vi "Cut-Out File Manager.vi"(6 "Local Data in":T1, 7 ".ini Controller":enum16{"Read", "Write"}(ring), 8 "error in (no error)":errorcluster, 11 "Run Path":path) -> (0 "error out":errorcluster, 4 "Local Data out":T1)   [LabVIEW 2024]
uses:
  Controls/Local Data.ctl
  Controls/Test Cluster.ctl
  Controls/Excluded Information.ctl
  Controls/Language.ctl
  <vilib>/Utility/file.llb/Write Delimited Spreadsheet (string).vi
  <vilib>/Utility/file.llb/Read Delimited Spreadsheet (string).vi
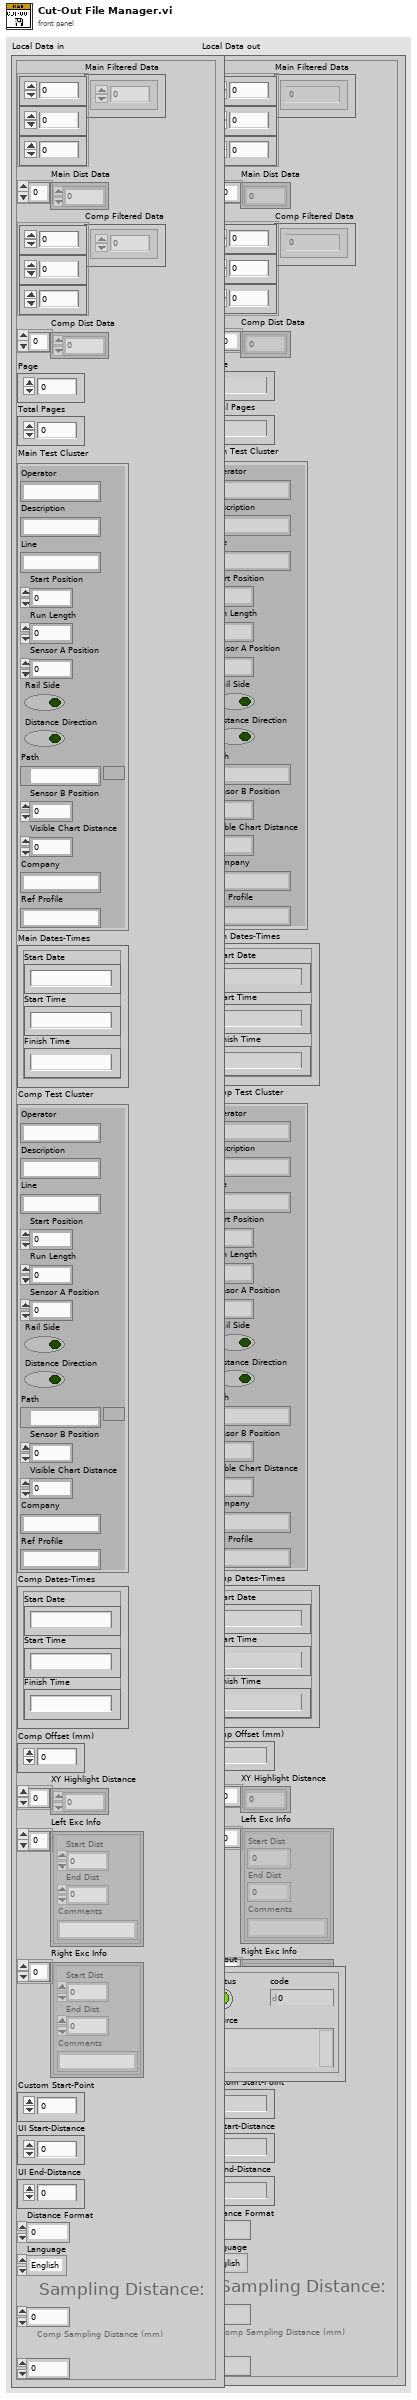
[diagram p1: front panel]
types:
  T1 = typedef "Local Data.ctl" = cluster{"Main Filtered Data":dbl[][][], "Main Dist Data":dbl[], "Comp Filtered Data":dbl[][][], "Comp Dist Data":dbl[], "Page":u8, "Total Pages":u8, "Main Test Cluster":T2, "Main Dates-Times":cluster{"Start Date":string, "Start Time":string, "Finish Time":string}, "Comp Test Cluster":T2, "Comp Dates-Times":cluster{"Start Date":string, "Start Time":string, "Finish Time":string}, "Comp Offset (mm)":i64, "XY Highlight Distance":dbl[], "Left Exc Info":T3[], "Right Exc Info":T3[], "Custom Start-Point":dbl, "UI Start-Distance":dbl, "UI End-Distance":dbl, "Distance Format":u8, "Language":T4, "Main Sampling Distance (mm)":dbl, "Comp Sampling Distance (mm)":dbl}
  T2 = typedef "Test Cluster.ctl" = cluster{"Operator":string, "Description":string, "Line":string, "Start Position":dbl, "Run Length":dbl, "Sensor A Position":dbl, "Rail Side":bool, "Distance Direction":bool, "Path":path, "Sensor B Position":dbl, "Visible Chart Distance":dbl, "Company":string, "Ref Profile":string}
  T3 = typedef "Excluded Information.ctl" = cluster{"Start Dist":dbl, "End Dist":dbl, "Comments":string}
  T4 = typedef "Language.ctl" = enum16{"English", "Chinese", "German"}
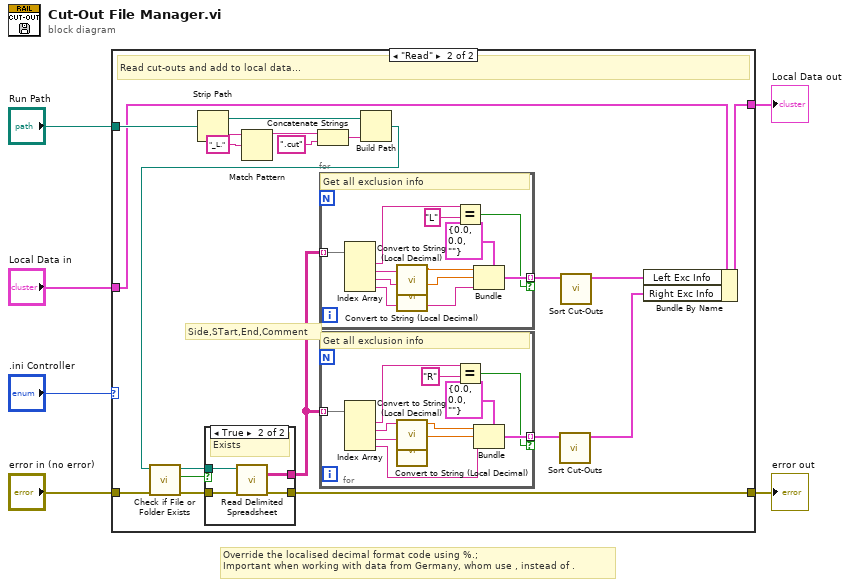
[diagram p0: block diagram]
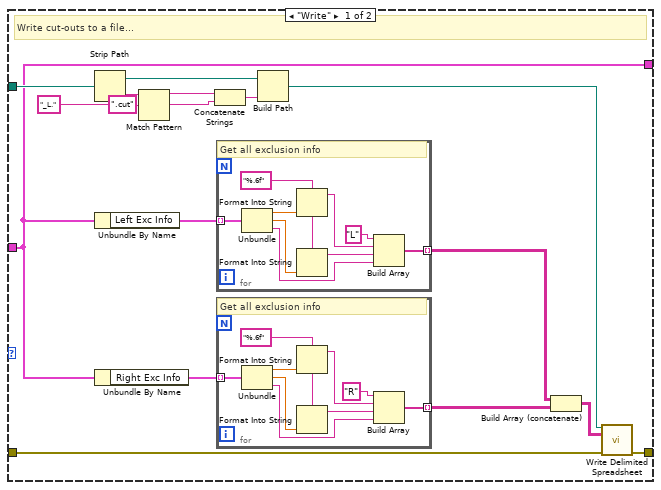
[diagram p2: hidden frame]
diagram:
  # "Override the localised decimal format code using %.;\nImportant when working with data from Germany, whom use , instead of ."
  n1 = case shown="\"Read\"" ".ini Controller" {
    tunnel: "Local Data in" -> [w9 w51]
    tunnel: "Run Path" -> [w15 w56]
    tunnel: "error in (no error)" -> [w11 w53]
    tunnel: [w10 w52] -> w4
    tunnel: [w9 w49] -> w6
    frame "Write" {
      # "Write cut-outs to a file..."
      n2 = Strip Path(path=w15) -> (stripped path=w14:path, name=w18:string)
      n3 = Unbundle By Name(w9) -> ("Left Exc Info"=w8:T3[])
      n4 = Unbundle By Name(w9) -> ("Right Exc Info"=w22:T3[])
      n5 = Match Pattern(string=w18, regular expression="_L.") -> (before substring=w17:string)  [unwired: 1 in, 3 out]
      n6 = Concatenate Strings(w17, ".cut" ("string")) -> (w13:string)
      n7 = for {
        tunnel: w8 -> [w31] mode=indexing
        tunnel: [w23] -> w7 mode=indexing
        w28 = "%.6f" ("format string")
        # "Get all exclusion info"
        n8 = Unbundle(w31) -> ("Start Dist"=w30:dbl, "End Dist"=w29:dbl, "Comments"=w25:string)
        n9 = Format Into String(format string=w28, w30) -> (resulting string=w27:string)  [unwired: 2 in, 1 out]
        n10 = Format Into String(format string=w28, w29) -> (resulting string=w26:string)  [unwired: 2 in, 1 out]
        n11 = Build Array("L" ("element"), w27, w26, w25) -> (w23:string[])
      }
      n12 = for {
        tunnel: w22 -> [w40] mode=indexing
        tunnel: [w32] -> w21 mode=indexing
        w37 = "%.6f" ("format string")
        # "Get all exclusion info"
        n13 = Unbundle(w40) -> ("Start Dist"=w39:dbl, "End Dist"=w38:dbl, "Comments"=w34:string)
        n14 = Format Into String(format string=w37, w39) -> (resulting string=w36:string)  [unwired: 2 in, 1 out]
        n15 = Format Into String(format string=w37, w38) -> (resulting string=w35:string)  [unwired: 2 in, 1 out]
        n16 = Build Array("R" ("element"), w36, w35, w34) -> (w32:string[])
      }
      n17 = Build Path(base path=w14, name or relative path=w13) -> (appended path=w12:path)
      n18 = Build Array (concatenate)(w7, w21) -> (w20:string[][])
      n19 = call-poly <vilib>:"Write Delimited Spreadsheet.vi"("file path (dialog if empty)"=w12, "2D data"=w20, "error in (no error)"=w11) -> ("error out"=w10:errorcluster)  [unwired: 11 in, 1 out]
    }
    frame "Read" {
      # "Side,STart,End,Comment"
      # "Read cut-outs and add to local data..."
      n20 = Strip Path(path=w56) -> (stripped path=w55:path, name=w59:string)
      n21 = Match Pattern(string=w59, regular expression="_L.") -> (before substring=w58:string)  [unwired: 1 in, 3 out]
      n22 = Concatenate Strings(w58, ".cut" ("string")) -> (w54:string)
      n23 = Build Path(base path=w55, name or relative path=w54) -> (appended path=w47:path)
      n24 = call <vilib>:"Check if File or Folder Exists.vi"("error in (no error)"=w53, "path"=w47) -> ("error out"=w48:errorcluster, "file or folder exists?"=w45:bool, "dup path"=w46:path)  [unwired: 7 in]
      n25 = case shown="True" w45 {
        tunnel: [w61 w65] -> w52
        tunnel: [_ w64] -> w50
        tunnel: w48 -> [w61 w63]
        tunnel: w46 -> [_ w62]
        frame False {
        }
        frame True {
          # "Exists"
          n26 = call-poly <vilib>:"Read Delimited Spreadsheet.vi"("file path (dialog if empty)"=w62, "error in (no error)"=w63) -> ("all rows"=w64:string[][], "error out"=w65:errorcluster)  [unwired: 8 in, 4 out]
        }
      }
      n27 = for {
        tunnel: w50 -> [w87] mode=indexing
        tunnel: [w83] -> w44 mode=indexing if=w82
        # "Get all exclusion info"
        n28 = Index Array(array=w87) -> (element #1=w85:string, element #2=w81:string, element #3=w78:string, element #4=w79:string)  [unwired: 4 in]
        n29 = call "Convert to String (Local Decimal).vi"("Distance (String)"=w81) -> ("Distance (DBL)"=w80:dbl)  [unwired: 10 in]
        n30 = call "Convert to String (Local Decimal).vi"("Distance (String)"=w78) -> ("Distance (DBL)"=w77:dbl)  [unwired: 10 in]
        n31 = Equal?(x=w85, y="L" ("element")) -> (x = y?=w82:bool)
        n32 = Bundle(cluster=T3 {"Start Dist"=0.0, "End Dist"=0.0, "Comments"=""}, "Start Dist"=w80, "End Dist"=w77, "Comments"=w79) -> (w83:T3)
      }
      n33 = for {
        tunnel: w50 -> [w76] mode=indexing
        tunnel: [w71] -> w42 mode=indexing if=w70
        # "Get all exclusion info"
        n34 = Index Array(array=w76) -> (element #1=w74:string, element #2=w69:string, element #3=w68:string, element #4=w72:string)  [unwired: 4 in]
        n35 = call "Convert to String (Local Decimal).vi"("Distance (String)"=w69) -> ("Distance (DBL)"=w66:dbl)  [unwired: 10 in]
        n36 = call "Convert to String (Local Decimal).vi"("Distance (String)"=w68) -> ("Distance (DBL)"=w67:dbl)  [unwired: 10 in]
        n37 = Equal?(x=w74, y="R" ("element")) -> (x = y?=w70:bool)
        n38 = Bundle(cluster=T3 {"Start Dist"=0.0, "End Dist"=0.0, "Comments"=""}, "Start Dist"=w66, "End Dist"=w67, "Comments"=w72) -> (w71:T3)
      }
      n39 = call "Sort Cut-Outs.vi"("Exc Info in"=w42) -> ("Exc Info out"=w41:T3[])  [unwired: 9 in, 1 out]
      n40 = call "Sort Cut-Outs.vi"("Exc Info in"=w44) -> ("Exc Info out"=w43:T3[])  [unwired: 9 in, 1 out]
      n41 = Bundle By Name(cluster=w51, "Left Exc Info"=w43, "Right Exc Info"=w41) -> (w49:T1)
    }
  }
  "Local Data out" <- w6
  "error out" <- w4
